vi "SGUI Example - demo 1.vi"() -> ()   [LabVIEW 2020, in "varilib.lvlib"]
doc: "SGUI lib demo 1. Basic usage of controls handling via SGUI library."
uses:
  varilib.lvlib
  SGUI Assign Multiple Strings With Tags By Label.vi
  SGUI Assign References Mode.ctl
  SGUI Set Single Integer By Label.vi
  SGUI Set Single Value and Uncertainty to String by Label.vi
panel:
  in  "unit":string
  in  "value":dbl=0.01112356 format="%#_7p"
  in  "uncertainty":dbl=4.56e-07 format="%#_6p"
  in  "caption":string="Programatically changed caption"
  out "value with uncertainty":string
  out "error out":errorcluster
  in  "btn stop":bool
  out "String 2":string caption="Programatically changed caption"
  out "String 1":string caption="String"
  out "Numeric":i32
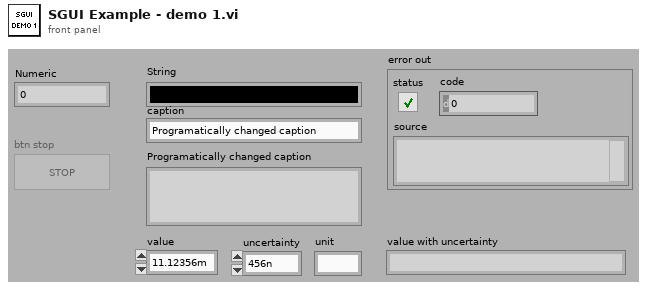
[diagram p1: front panel]
types:
  T1 = typedef "varilib.lvlib/SGUI Assign References Mode.ctl" = enum16{"Add to stack", "Overwrite", "Release last", "Release ID"}
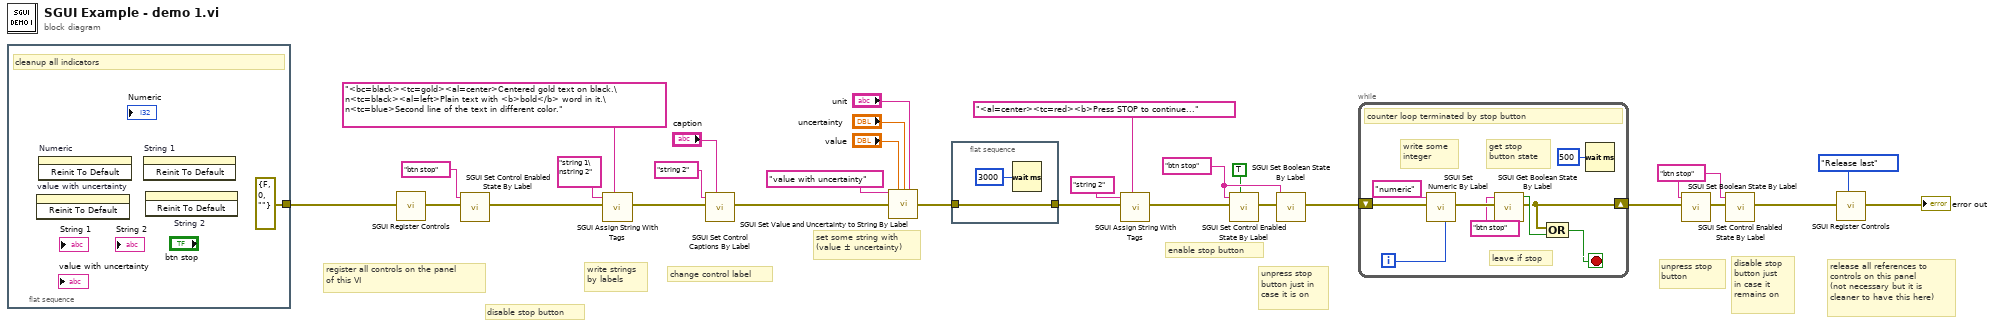
[diagram p0: block diagram]
diagram:
  w15 = "btn stop" ("control label ('btn stop')")
  w22 = "btn stop" ("control label ('btn stop')")
  # "set some string with\n(value ± uncertainty)"
  # "release all references to\ncontrols on this panel\n(not necessary but it is\ncleaner to have this here)"
  # "disable stop\nbutton just\nin case it\nremains on"
  # "disable stop button"
  # "enable stop button"
  # "unpress stop\nbutton"
  # "unpress stop\nbutton just in\ncase it is on"
  # "change control label"
  # "write strings\nby labels"
  # "register all controls on the panel\nof this VI"
  n1 = flat-sequence {
    tunnel: [errorcluster {"status"=FALSE, "code"=0, "source"=""} ("error out")] -> w8
    frame #0 {
      # "cleanup all indicators"
      n2 = invoke on="value with uncertainty" class="Str" method="Reinit To Default"() -> ()  [unwired: 3 in, 3 out]
      n3 = invoke on="Numeric" class="DigNum (strict)" method="Reinit To Default"() -> ()  [unwired: 3 in, 3 out]
      n4 = invoke on="String 1" class="Str" method="Reinit To Default"() -> ()  [unwired: 3 in, 3 out]
      n5 = invoke on="String 2" class="Str" method="Reinit To Default"() -> ()  [unwired: 3 in, 3 out]
    }
  }
  n6 = call "SGUI Register Controls.vi"("error in"=w8) -> ("error out"=w19:errorcluster)  [unwired: 16 in, 2 out]
  n7 = call "SGUI Set Control Enabled State By Label.vi"("error in"=w19, "labels (empty)"="btn stop") -> ("error out"=w18:errorcluster)  [unwired: 8 in, 1 out]
  n8 = call-poly "SGUI Assign String With Tags.vi"("error in"=w18, "label(s) (empty)"="string 1\nstring 2" ("string (empty)"), "string (empty)"="<bc=black><tc=gold><al=center>Centered gold text on black.\n<tc=black><al=left>Plain text with <b>bold</b> word in it.\n<tc=blue>Second line of the text in different color.") -> ("error out"=w26:errorcluster)  [unwired: 7 in, 1 out]
  n9 = call "SGUI Set Control Captions By Label.vi"("error in"=w26, "labels (empty)"="string 2" ("captions (empty)"), "captions (empty)"="caption") -> ("error out"=w6:errorcluster)  [unwired: 7 in, 1 out]
  n10 = call-poly "SGUI Set Value and Uncertainty to String By Label.vi"("label (empty)"="value with uncertainty", "value (empty)"="value", "uncertainty (empty)"="uncertainty", "unit (empty)"="unit", "error in"=w6) -> ("error out"=w5:errorcluster)  [unwired: 9 in, 1 out]
  n11 = flat-sequence {
    tunnel: [w32] -> w13
    tunnel: w5 -> [w32]
    frame #0 {
      n12 = Wait (ms)(milliseconds to wait=u32 3000) -> ()  [unwired: 1 out]
    }
  }
  n13 = call-poly "SGUI Assign String With Tags.vi"("error in"=w13, "label(s) (empty)"="string 2", "string (empty)"="<al=center><tc=red><b>Press STOP to continue...") -> ("error out"=w12:errorcluster)  [unwired: 7 in, 1 out]
  n14 = call "SGUI Set Control Enabled State By Label.vi"("error in"=w12, "labels (empty)"=w22, "Enabled? (False)"=TRUE) -> ("error out"=w20:errorcluster)  [unwired: 7 in, 1 out]
  n15 = call "SGUI Set Boolean State By Label.vi"("error in"=w20, "control label(s) ('btn stop')"=w22) -> ("error out"=w24:errorcluster)  [unwired: 8 in, 1 out]
  n16 = while {
    shift-right: [w36] -> w23
    shift-left: w24 -> [w41]
    i -> [w33]
    stop <- w38 stop-if-true
    # "leave if stop"
    # "get stop\nbutton state"
    # "write some\ninteger"
    # "counter loop terminated by stop button"
    n17 = call-poly "SGUI Set Numeric By Label.vi"("error in"=w41, "label (empty)"="numeric", "value (none)"=w33) -> ("error out"=w39:errorcluster)  [unwired: 7 in, 1 out]
    n18 = call "SGUI Get Boolean State By Label.vi"("error in"=w39, "control label ('btn stop')"="btn stop") -> ("error out"=w36:errorcluster, "binary state out"=w37:bool)  [unwired: 7 in, 1 out]
    n19 = Compound Arithmetic op=OR(w36, w37) -> (w38:bool)
    n20 = Wait (ms)(milliseconds to wait=u32 500) -> ()  [unwired: 1 out]
  }
  n21 = call "SGUI Set Boolean State By Label.vi"("error in"=w23, "control label(s) ('btn stop')"=w15) -> ("error out"=w16:errorcluster)  [unwired: 8 in, 1 out]
  n22 = call "SGUI Set Control Enabled State By Label.vi"("error in"=w16, "labels (empty)"=w15) -> ("error out"=w14:errorcluster)  [unwired: 8 in, 1 out]
  n23 = call "SGUI Register Controls.vi"("error in"=w14, "register mode (overwrite)"=SGUI_Assign_References_Mode."Release last") -> ("error out"=→"error out":errorcluster)  [unwired: 15 in, 2 out]
